vi "Process.vi"(8 "error in":errorcluster, 11 "Logger":refnum<class "Logger.lvclass">) -> (0 "error out":errorcluster, 3 "Logger out":refnum<class "Logger.lvclass">)   [LabVIEW 2019, in "Logger.lvlib" / "Logger.lvclass"]
doc: "---------------------------------------------------------------\nJKI State Machine Objects™\nhttp://jki.net/state-machine-objects/\nCopyright (C) 2005-2015, JKI <info@jki.net>\nALL RIGHTS RESERVED"
uses:
  Logger.lvclass
  C:/Program Files (x86)/National Instruments/LabVIEW 2019/vi.lib/JKI/JKI SMO/smo.lvlibp/SMO/SMO.lvclass
  <vilib>/JKI/JKI SMO/smo.lvlibp/SMO/SMO.lvclass
  <userlib>/LevyLab/Debug/Debug.lvlib
panel:
  out "String":string
  # "For instructions on how to use the JKI State Machine Objects, examples and video tutorials, visit:\nhttp://jki.net/state-machine-objects/\n\nJKI State Machine Objects™\nhttp://jki.net/state-machine-objects/\nCopyright (C) 2005-2015, JKI <info@jki.net>\nALL RIGHTS RESERVED"
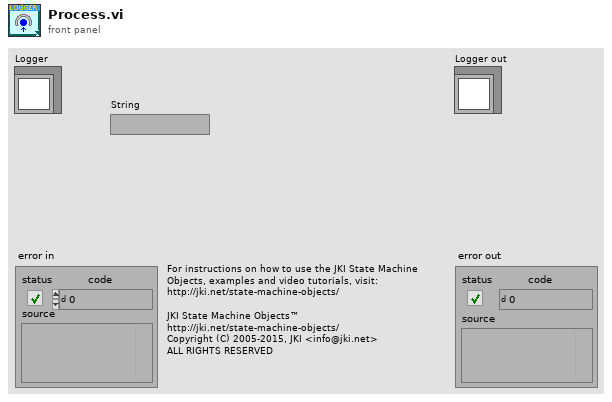
[diagram p1: front panel]
types:
  T1 = enum32{"invalid app kind", "Development System", "Run Time System", "Student Edition", "Embedded LabVIEW", "Evaluation", "Custom"}
  T2 = enum32{"Invalid", "Standard", "Closed", "Hidden", "Minimized", "Maximized"}
  T3 = cluster{"Core":cluster{"Current VI Reference":refnum<vi>, "Close Panel on Exit?":bool, "Last Error":cluster{"error":errorcluster, "previous state":string, "remaining states":string}, "Shutdown?":bool}, "SelfRef":refnum<class "Logger.lvclass">}
  T4 = cluster{"Current VI Reference":refnum<vi>, "Close Panel on Exit?":bool, "Last Error":cluster{"error":errorcluster, "previous state":string, "remaining states":string}, "Shutdown?":bool}
  T5 = typedef "Debug.lvlib/Attribute.Debug.lvclass/DebugBehavior.ctl" = enum16{"Normal", "Debug"}
  T6 = typedef "smo.lvlibp/SMO.lvclass/Protected Events.ctl" = cluster{"StopProcesses":refnum<user-event>, "AbortProcesses":refnum<user-event>, "Config Changed":refnum<user-event>, "Dependency":refnum<user-event>}
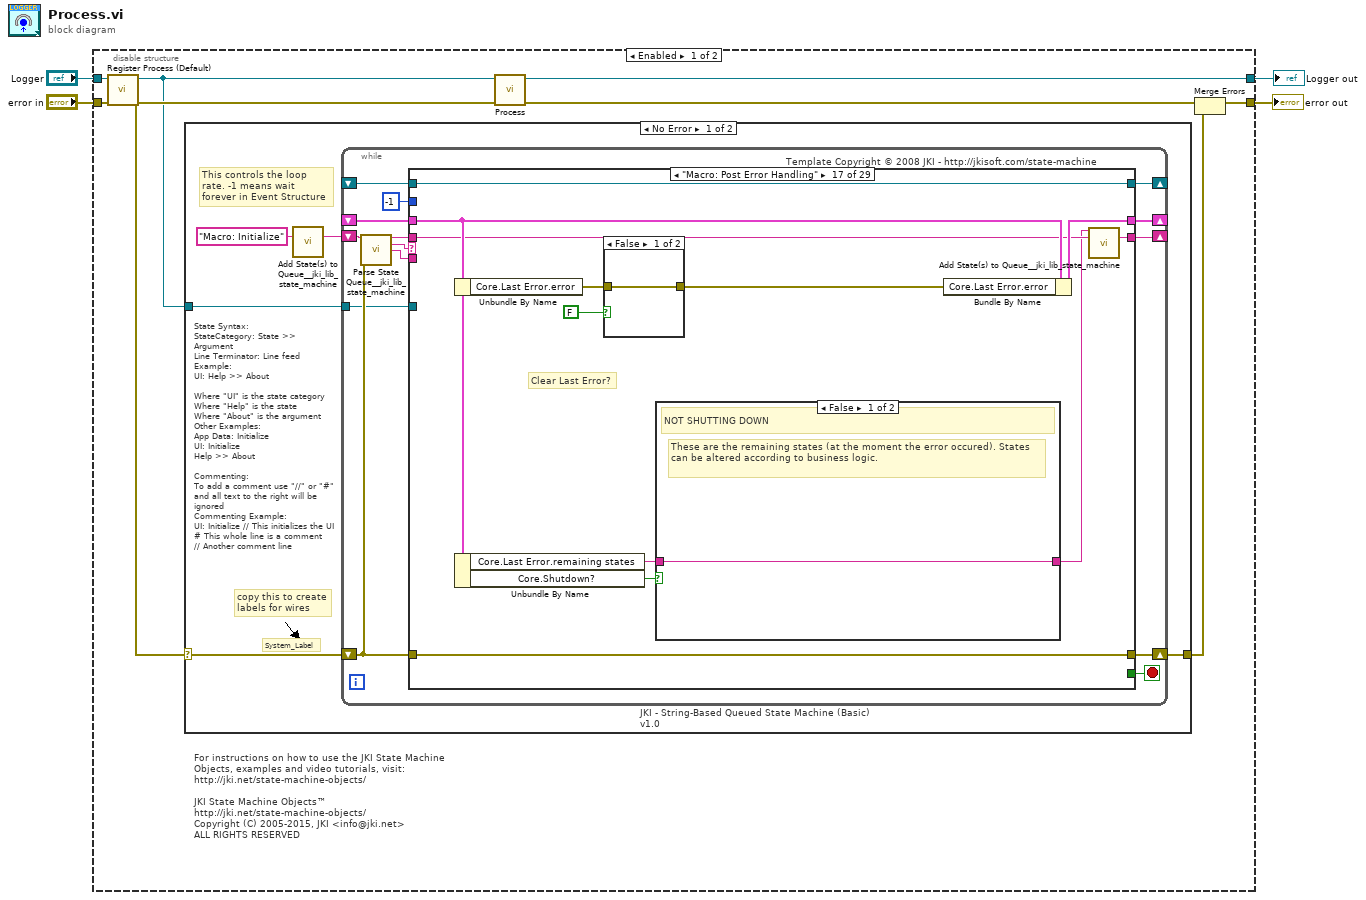
[diagram p0: block diagram]
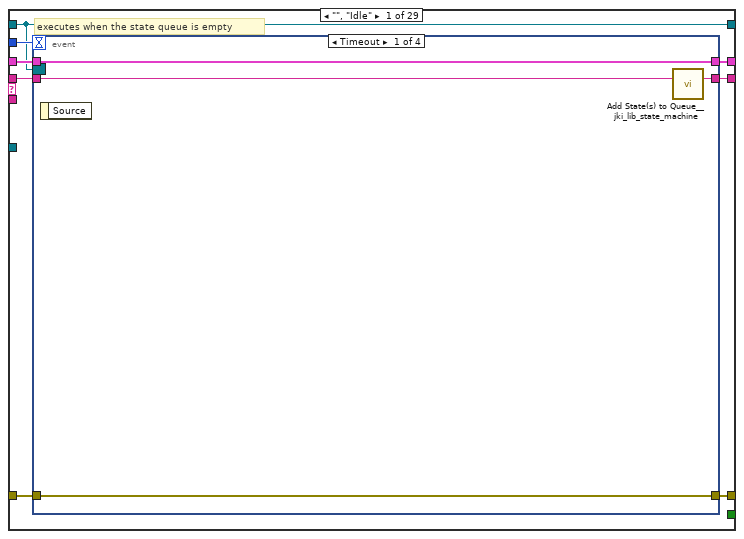
[diagram p2: hidden frame]
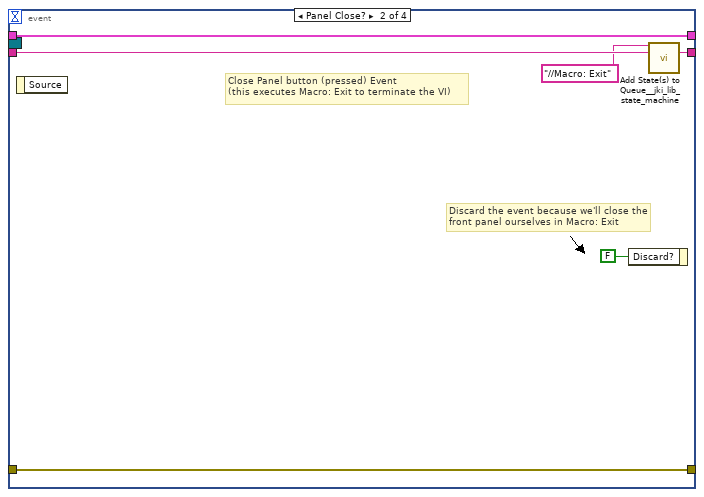
[diagram p3: hidden frame]
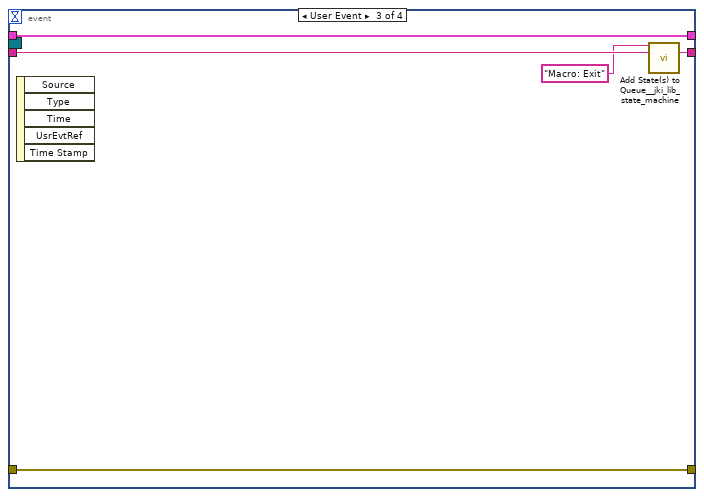
[diagram p4: hidden frame]
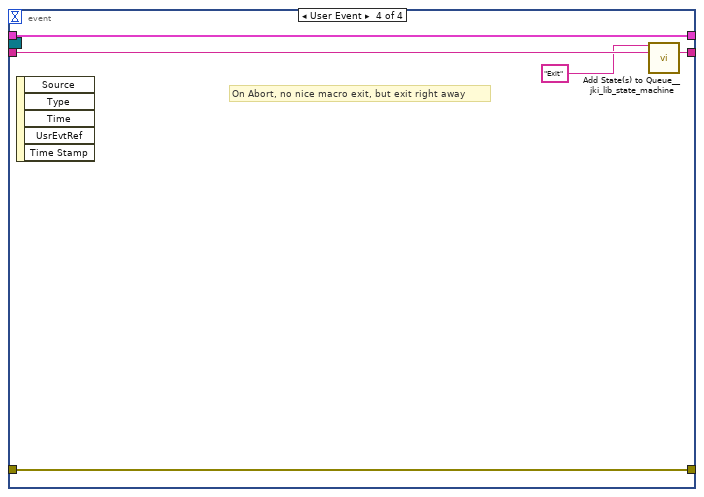
[diagram p5: hidden frame]
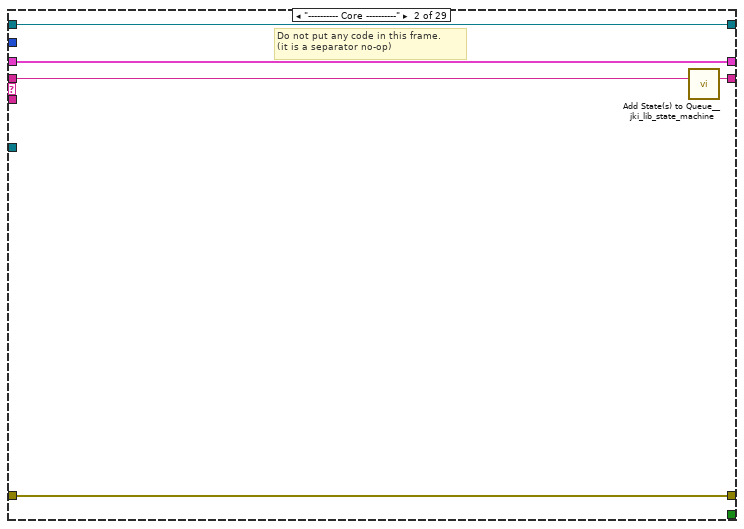
[diagram p6: hidden frame]
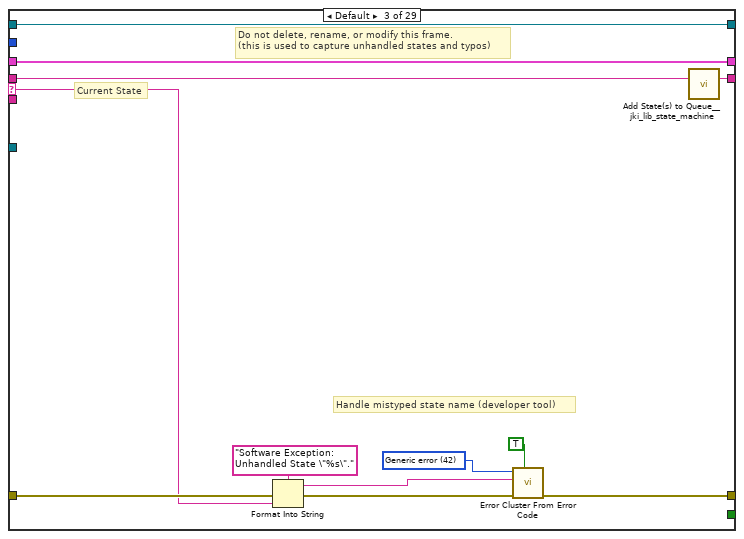
[diagram p7: hidden frame]
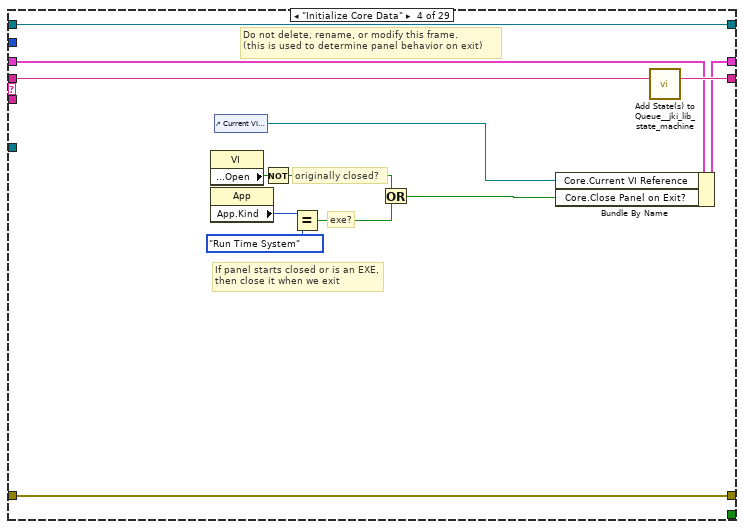
[diagram p8: hidden frame]
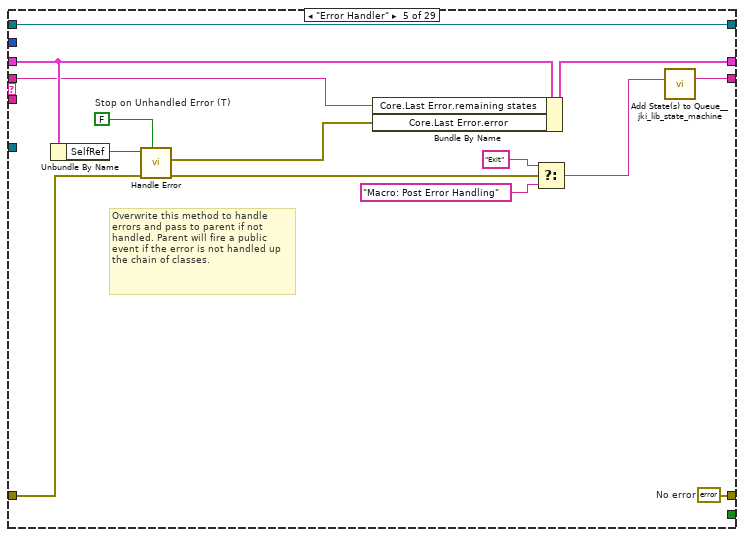
[diagram p9: hidden frame]
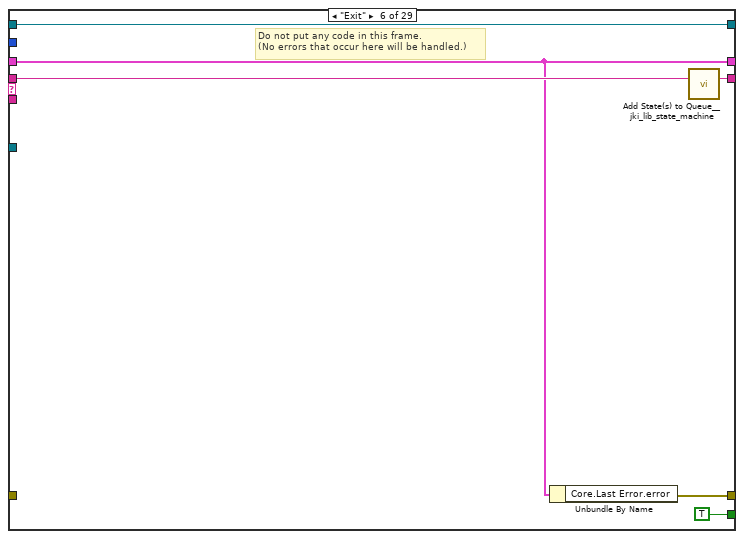
[diagram p10: hidden frame]
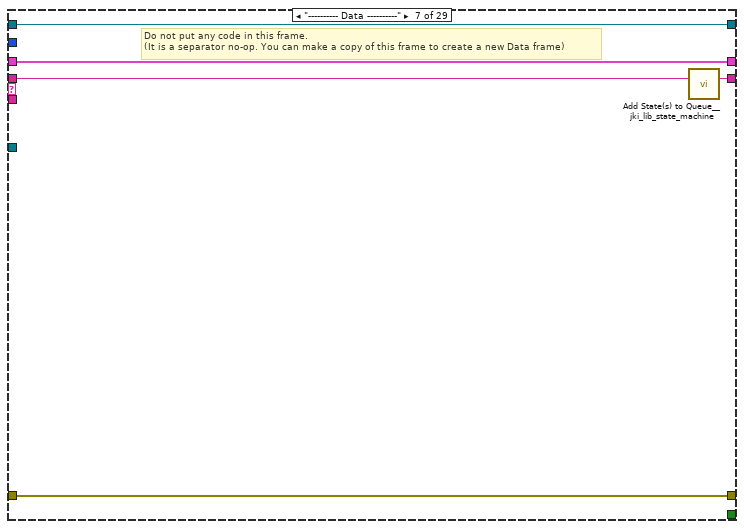
[diagram p11: hidden frame]
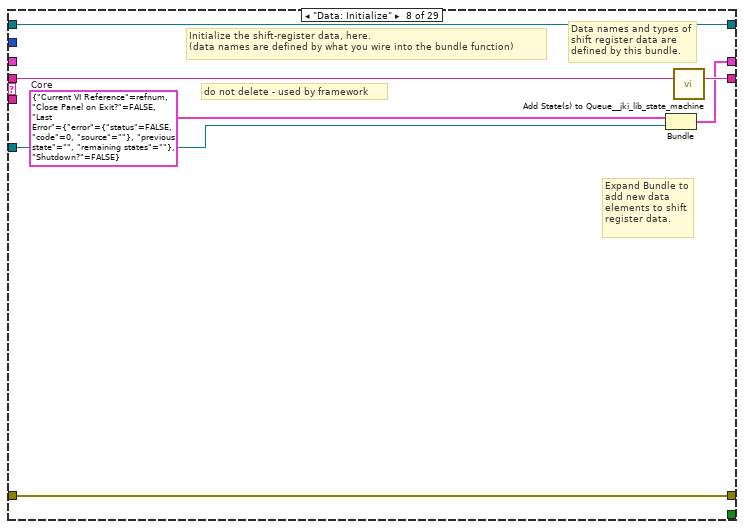
[diagram p12: hidden frame]
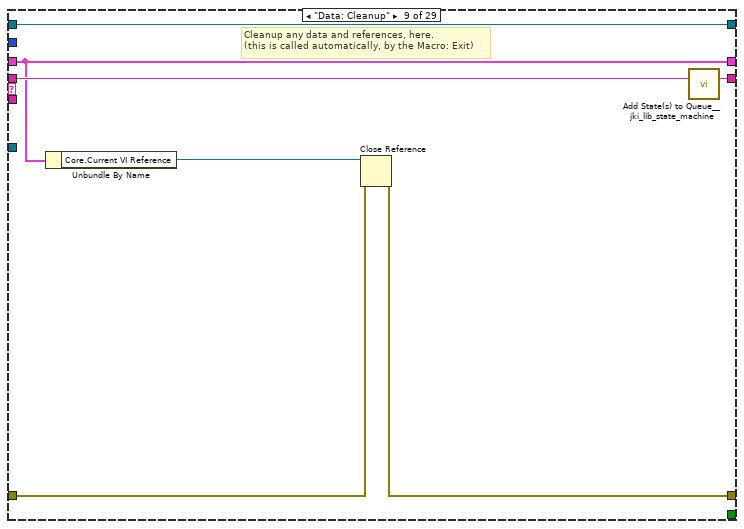
[diagram p13: hidden frame]
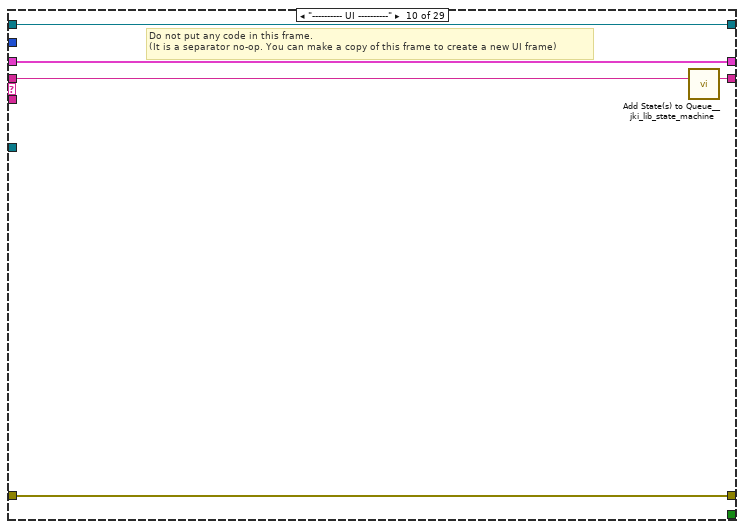
[diagram p14: hidden frame]
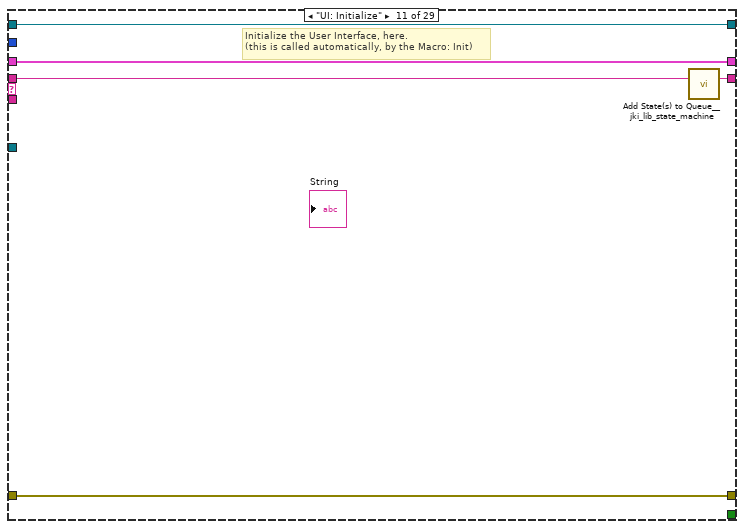
[diagram p15: hidden frame]
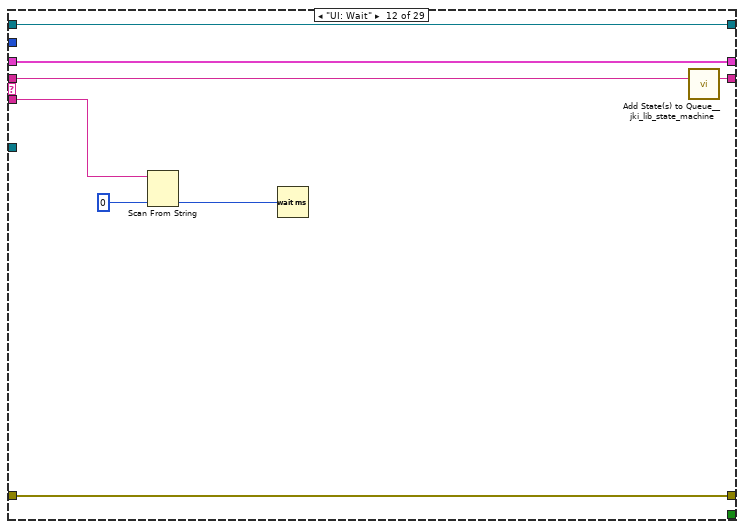
[diagram p16: hidden frame]
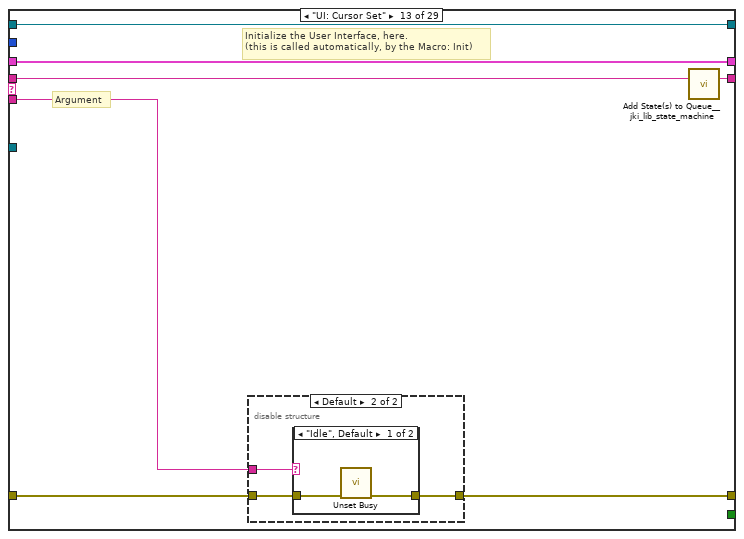
[diagram p17: hidden frame]
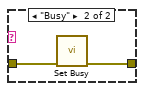
[diagram p19: hidden frame]
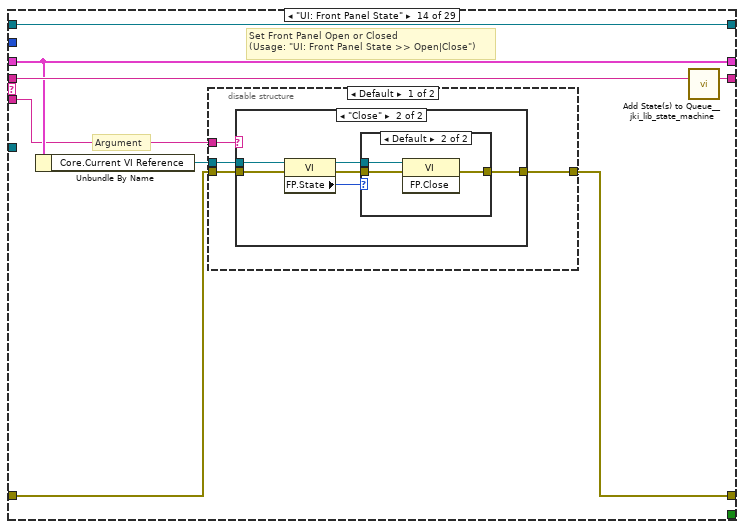
[diagram p20: hidden frame]
diagram:
  n1 = disable-structure shown="Enabled" {
    disable-tunnel: "Logger" -> [w12 w336]
    disable-tunnel: "error in" -> [w11 w335]
    disable-tunnel: [w10 w335] -> w2
    disable-tunnel: [w7 w336] -> w1
    frame Enabled {
      # "For instructions on how to use the JKI State Machine Objects, examples and video tutorials, visit:\nhttp://jki.net/state-machine-objects/\n\nJKI State Machine Objects™\nhttp://jki.net/state-machine-objects/\nCopyright (C) 2005-2015, JKI <info@jki.net>\nALL RIGHTS RESERVED"
      n2 = call <vilib>:"Register Process (Default).vi"("error in (no error)"=w11, "SMO"=w12) -> ("error out"=w9:errorcluster, "SelfRef"=w8:refnum<class "Logger.lvclass">)  [unwired: 8 in]
      n3 = case shown="No Error" w9 {
        selector: w9 -> [w14 w334]
        tunnel: w8 -> [w15 _]
        tunnel: [w13 w334] -> w5
        frame No Error {
          # "State Syntax:\nStateCategory: State >> Argument\nLine Terminator: Line feed\nExample:\nUI: Help >> About\n\nWhere \"UI\" is the state category\nWhere \"Help\" is the state\nWhere \"About\" is the argument\nOther Examples:\nApp Data: Initialize\nUI: Initialize\nHelp >> About\n\nCommenting:\nTo add a comment use \"//\" or \"#\" and all text to the right will be ignored\nCommenting Example:\nUI: Initialize // This initializes the UI\n# This whole line is a comment\n// Another comment line"
          # "copy this to create labels for wires"
          # "This controls the loop rate. -1 means wait forever in Event Structure"
          # "System_Label"
          n4 = call <vilib>:"Add State(s) to Queue__jki_lib_state_machine.vi"("State(s) in (\"\")"="Macro: Initialize") -> ("States Out"=w17:string)  [unwired: 14 in]
          n5 = while "JKI - String-Based Queued State Machine (Basic) v1.0" {
            shift-right: [w19] -> _
            shift-left: _ -> [w18]
            shift-right: [w27] -> w13
            shift-left: w14 -> [w23]
            shift-right: [w26] -> _
            shift-left: w17 -> [w28]
            tunnel: w15 -> [w22]
            shift-right: [w21] -> _
            shift-left: _ -> [w20]
            stop <- w25 stop-if-true
            # "Template Copyright © 2008 JKI - http://jkisoft.com/state-machine"
            n6 = call <vilib>:"Parse State Queue__jki_lib_state_machine.vi"("State Queue"=w28, "Error In (no error)"=w23) -> ("Remaining States"=w30:string, "Current State"=w31:string, "Arguments"=w29:string)  [unwired: 11 in]
            n7 = case shown="\"Macro: Post Error Handling\"" w31 {
              selector: w31 -> [_ _ w66 _ _ _ _ _ _ _ _ _ _ _ _ _ _ _ _ _ _ _ _ _ _ _ _ _ _]
              tunnel: w30 -> [w39 w64 w70 w89 w92 w109 w114 w121 w128 w133 w138 w146 w153 w169 w201 w213 w215 w244 w265 w270 w281 w286 w296 w302 w307 w316 w321 w326 w333]
              tunnel: w29 -> [_ _ _ _ _ _ _ _ _ _ _ w139 w147 w163 _ _ _ _ _ _ _ _ _ _ _ _ _ _ _]
              tunnel: w18 -> [w37 w61 w68 w80 w93 w105 w111 _ w123 w130 w136 w143 w151 w165 w198 w206 w216 w232 w251 w267 w271 w283 w294 w300 w305 w313 w317 w322 w330]
              tunnel: [w36 w62 w72 w86 w99 w104 w112 w115 w124 w131 w135 w144 w148 w166 w199 w202 w224 w231 w263 w268 w273 w284 w289 w298 w303 w308 w318 w323 w327] -> w27
              tunnel: w23 -> [w35 w62 w71 w86 w100 _ w112 w115 w125 w131 w135 w144 w149 w167 w199 w202 w224 w230 w263 w268 w274 w284 w290 w298 w303 w309 w318 w323 w328]
              tunnel: [w38 w63 w69 w88 w103 w108 w113 w120 w127 w132 w137 w145 w152 w168 w200 w212 w225 w243 w264 w269 w280 w285 w295 w301 w306 w315 w320 w325 w332] -> w26
              tunnel: [_ _ _ _ _ TRUE _ _ _ _ _ _ _ _ _ _ _ _ _ _ _ _ _ _ _ _ _ _ _] -> w25
              tunnel: [w34 w61 w68 w87 w98 w105 w111 w117 w123 w130 w136 w143 w151 w165 w198 w206 w217 w234 w252 w267 w271 w283 w294 w300 w305 w312 w317 w322 w330] -> w19
              tunnel: -1 ("Timeout") -> [w33 _ _ _ _ _ _ _ _ _ _ _ _ _ _ _ _ _ _ _ _ _ _ _ _ _ _ _ _]
              tunnel: w22 -> [_ _ _ _ _ _ _ w116 _ _ _ _ _ _ _ _ _ _ _ _ _ _ _ _ _ _ _ _ _]
              tunnel: [w32 w60 w65 w77 w102 w106 w110 w119 w122 w129 w134 w142 w150 w162 w197 w211 w223 w242 w258 w266 w279 w282 w293 w299 w304 w314 w319 w324 w331] -> w21
              tunnel: w20 -> [w32 w60 w65 w77 w102 w106 w110 w119 w122 w129 w134 w142 w150 w162 w197 w211 w223 w242 w258 w266 w279 w282 _ w299 w304 w314 w319 w324 w331]
              frame "", "Idle" {
                # "executes when the state queue is empty"
                n8 = event shown="[0] Timeout" {
                  selector: w32 -> [_ _ _ _]
                  dyn-events: _ -> [_ _ _ _]
                  timeout: w33 -> [_ _ _ _]
                  tunnel: w39 -> [w43 w49 w54 w59]
                  tunnel: [w42 w48 w53 w58] -> w38
                  tunnel: w37 -> [w41 w46 w51 w56]
                  tunnel: [w40 w47 w52 w57] -> w36
                  tunnel: w35 -> [w40 w47 w52 w57]
                  tunnel: [w41 w46 w51 w56] -> w34
                  event Timeout {
                    n9 = event-data() -> ()  [unwired: 1 in, 1 out]
                    n10 = call <vilib>:"Add State(s) to Queue__jki_lib_state_machine.vi"("State(s) in (\"\")"=w43) -> ("States Out"=w42:string)  [unwired: 14 in]
                  }
                  event Panel Close? {
                    # "Discard the event because we'll close the front panel ourselves in Macro: Exit"
                    # "Close Panel button (pressed) Event\n(this executes Macro: Exit to terminate the VI)"
                    n11 = event-data() -> ()  [unwired: 1 in, 1 out]
                    n12 = event-data("Discard?"=FALSE) -> ()  [unwired: 1 in, 1 out]
                    n13 = call <vilib>:"Add State(s) to Queue__jki_lib_state_machine.vi"("State(s) in Front (\"\")"="//Macro: Exit", "State(s) in (\"\")"=w49) -> ("States Out"=w48:string)  [unwired: 13 in]
                  }
                  event User Event {
                    n14 = event-data() -> ()  [unwired: 1 in, 5 out]
                    n15 = call <vilib>:"Add State(s) to Queue__jki_lib_state_machine.vi"("State(s) in Front (\"\")"="Macro: Exit", "State(s) in (\"\")"=w54) -> ("States Out"=w53:string)  [unwired: 13 in]
                  }
                  event User Event {
                    # "On Abort, no nice macro exit, but exit right away"
                    n16 = event-data() -> ()  [unwired: 1 in, 5 out]
                    n17 = call <vilib>:"Add State(s) to Queue__jki_lib_state_machine.vi"("State(s) in Front (\"\")"="Exit", "State(s) in (\"\")"=w59) -> ("States Out"=w58:string)  [unwired: 13 in]
                  }
                }
              }
              frame "---------- Core ----------" {
                # "Do not put any code in this frame.\n(it is a separator no-op)"
                n18 = call <vilib>:"Add State(s) to Queue__jki_lib_state_machine.vi"("State(s) in (\"\")"=w64) -> ("States Out"=w63:string)  [unwired: 14 in]
              }
              frame Default {
                w75 = 42 items=["No error", "Argument error", "Memory is full", "Out of zone", "End of file", "File already open", "Generic file I/O error", "File not found", "File permission error", "Disk is full", "Duplicate path", "Too many files open", "System feature not enabled", "Resource file not found", "Cannot add resource", "Resource not found", "Image not found", "Image memory error", "Pen does not exist", "Config type invalid", "Config token not found", "Config parse error", "Config memory error", "Bad external code format", "Bad external code offset", "External code not present", "Null window", "Destroy window error", "Null menu", "Print aborted", "Bad print record", "Print driver error", "Windows error during printing", "Memory error during printing", "Print dialog error", "Generic print error", "Invalid device refnum", "Device not found", "Device parameter error", "Device unit error", "Cannot open device", "Device call aborted", "Generic error", "Cancelled by user", "Object ID too low", "Object ID too high", "Object not in heap", "Unknown heap", "Unknown object (invalid DefProc)", "Unknown object (DefProc not in table)", "Message out of range", "Invalid (null) method", "Unknown message", "Manager call not supported", "Bad address", "Network operation in progress", "Network operation timed out", "Connection is busy", "Network attribute not supported", "Network error", "Address in use", "System out of memory", "Connection aborted", "Connection refused", "Not connected", "Already connected", "Connection closed", "Initialization error (interapplication manager)", "Bad occurrence", "Wait on unbound occurrence handler", "Occurrence queue overflow", "Datalog type conflict", "Unused", "Unrecognized type (interapplication manager)", "Memory corrupt", "Failed to make temporary DLL", "Old CIN version", "Drag socket not found", "Failed to load drop-object", "Failed to register OLE object", "Failed to release OLE object", "Format specifier type mismatch", "Unknown format specifier", "Too few format specifiers", "Too many format specifiers", "Scan failed", "Newer CIN version", "Error converting to variant", "Runtime menu error", "Password tampered", "Variant attribute not found", "Incompatible variant data type", "Event data is not available", "Event Store is not present", "Occurrence is not found", "Event Queue is not created", "Event info is not available", "Refnum passed is NULL", "Error retrieving Class GUID", "Error retrieving CoClass GUID", "Error retrieving TypeLib GUID.", "Bad built application magic bytes.", "Specific driver is different from the specific driver associated with the Logical Name.", "There is no session opened to the class driver.", "Max Error", "MAX - Error with config objects", "MAX - Error loading configuration", "MAX - Group not supported"]
                # "Current State"
                # "Do not delete, rename, or modify this frame.\n(this is used to capture unhandled states and typos)"
                # "Handle mistyped state name (developer tool)"
                n19 = Format Into String(format string="Software Exception: Unhandled State \"%s\"." ("message"), error in=w71, w66) -> (resulting string=w74:string, error out=w73:errorcluster)  [unwired: 1 in]
                n20 = call <vilib>:"Error Cluster From Error Code.vi"("show call chain? (False)"=TRUE, "error in (no error)"=w73, "error message (\"\")"=w74, "error code (0)"=w75) -> ("error out"=w72:errorcluster)  [unwired: 5 in]
                n21 = call <vilib>:"Add State(s) to Queue__jki_lib_state_machine.vi"("State(s) in (\"\")"=w70) -> ("States Out"=w69:string)  [unwired: 14 in]
              }
              frame "Initialize Core Data" {
                # "Do not delete, rename, or modify this frame.\n(this is used to determine panel behavior on exit)"
                # "originally closed?"
                # "exe?"
                # "If panel starts closed or is an EXE, then close it when we exit"
                n22 = property class="VI"() -> ("Front Panel.Open"=w85:bool)  [unwired: 2 in, 2 out]
                n23 = property class="App"() -> ("App.Kind"=w84:T1)  [unwired: 2 in, 2 out]
                n24 = control-ref of="Current VI Reference"() -> (w78:refnum<vi>)
                n25 = Not(x=w85) -> (.not. x?=w82:bool)
                n26 = Equal?(x=w84, y=T1."Run Time System" ("Application:Kind")) -> (x = y?=w81:bool)
                n27 = Or(x=w82, y=w81) -> (x .or. y?=w79:bool)
                n28 = Bundle By Name(cluster=w80, "Core.Current VI Reference"=w78, "Core.Close Panel on Exit?"=w79) -> (w87:T3)
                n29 = call <vilib>:"Add State(s) to Queue__jki_lib_state_machine.vi"("State(s) in (\"\")"=w89) -> ("States Out"=w88:string)  [unwired: 14 in]
              }
              frame "Error Handler" {
                w94 = FALSE  # Stop on Unhandled Error (T)
                w99 = errorcluster {"status"=FALSE, "code"=0, "source"=""}  # No error
                # "Overwrite this method to handle errors and pass to parent if not handled. Parent will fire a public event if the error is not handled up the chain of classes."
                n30 = Unbundle By Name(w93) -> ("SelfRef"=w101:refnum<class "Logger.lvclass">)
                n31 = call-dynamic "Handle Error.vi"("Stop on Unhandled Error (T)"=w94, "error in"=w100, "SMO"=w101) -> ("handling error"=w95:errorcluster, "Unhandled error"=w97:errorcluster)  [unwired: 6 in, 1 out]
                n32 = Bundle By Name(cluster=w93, "Core.Last Error.remaining states"=w92, "Core.Last Error.error"=w97) -> (w98:T3)
                n33 = Select(t="Exit", s=w95, f="Macro: Post Error Handling") -> (s? t:f=w90:string)
                n34 = call <vilib>:"Add State(s) to Queue__jki_lib_state_machine.vi"("State(s) in (\"\")"=w90) -> ("States Out"=w103:string)  [unwired: 14 in]
              }
              frame "Exit" {
                # "Do not put any code in this frame.\n(No errors that occur here will be handled.)"
                n35 = Unbundle By Name(w105) -> ("Core.Last Error.error"=w104:errorcluster)
                n36 = call <vilib>:"Add State(s) to Queue__jki_lib_state_machine.vi"("State(s) in (\"\")"=w109) -> ("States Out"=w108:string)  [unwired: 14 in]
              }
              frame "---------- Data ----------" {
                # "Do not put any code in this frame.\n(It is a separator no-op. You can make a copy of this frame to create a new Data frame)"
                n37 = call <vilib>:"Add State(s) to Queue__jki_lib_state_machine.vi"("State(s) in (\"\")"=w114) -> ("States Out"=w113:string)  [unwired: 14 in]
              }
              frame "Data: Initialize" {
                w118 = T4 {"Current VI Reference"=refnum, "Close Panel on Exit?"=FALSE, "Last Error"={"error"={"status"=FALSE, "code"=0, "source"=""}, "previous state"="", "remaining states"=""}, "Shutdown?"=FALSE}  # Core
                # "do not delete - used by framework"
                # "Expand Bundle to add new data elements to shift register data."
                # "Data names and types of shift register data are defined by this bundle."
                # "Initialize the shift-register data, here.\n(data names are defined by what you wire into the bundle function)"
                n38 = Bundle("Core"=w118, "SelfRef"=w116) -> (w117:T3)  [unwired: 1 in]
                n39 = call <vilib>:"Add State(s) to Queue__jki_lib_state_machine.vi"("State(s) in (\"\")"=w121) -> ("States Out"=w120:string)  [unwired: 14 in]
              }
              frame "Data: Cleanup" {
                # "Cleanup any data and references, here.\n(this is called automatically, by the Macro: Exit)"
                n40 = Unbundle By Name(w123) -> ("Core.Current VI Reference"=w126:refnum<vi>)
                n41 = Close Reference(reference=w126, error in (no error)=w125) -> (error out=w124:errorcluster)
                n42 = call <vilib>:"Add State(s) to Queue__jki_lib_state_machine.vi"("State(s) in (\"\")"=w128) -> ("States Out"=w127:string)  [unwired: 14 in]
              }
              frame "---------- UI ----------" {
                # "Do not put any code in this frame.\n(It is a separator no-op. You can make a copy of this frame to create a new UI frame)"
                n43 = call <vilib>:"Add State(s) to Queue__jki_lib_state_machine.vi"("State(s) in (\"\")"=w133) -> ("States Out"=w132:string)  [unwired: 14 in]
              }
              frame "UI: Initialize" {
                # "Initialize the User Interface, here.\n(this is called automatically, by the Macro: Init)"
                n44 = call <vilib>:"Add State(s) to Queue__jki_lib_state_machine.vi"("State(s) in (\"\")"=w138) -> ("States Out"=w137:string)  [unwired: 14 in]
              }
              frame "UI: Wait" {
                n45 = Scan From String(input string=w139, default 1=u32 0) -> (output 1=w140:u32)  [unwired: 3 in, 3 out]
                n46 = Wait (ms)(milliseconds to wait=w140) -> ()  [unwired: 1 out]
                n47 = call <vilib>:"Add State(s) to Queue__jki_lib_state_machine.vi"("State(s) in (\"\")"=w146) -> ("States Out"=w145:string)  [unwired: 14 in]
              }
              frame "UI: Cursor Set" {
                # "Argument"
                # "Initialize the User Interface, here.\n(this is called automatically, by the Macro: Init)"
                n48 = disable-structure shown="Default" {
                  disable-tunnel: w149 -> [w154 w157]
                  disable-tunnel: [w154 w156] -> w148
                  disable-tunnel: w147 -> [_ w155]
                  frame condition #0 {
                  }
                  frame condition #1 (active) {
                    n49 = case shown="\"Idle\", Default" w155 {
                      tunnel: w157 -> [w159 w161]
                      tunnel: [w158 w160] -> w156
                      frame "Idle", Default {
                        n50 = call <vilib>:"Unset Busy.vi"("error in (no error)"=w159) -> ("error out"=w158:errorcluster)  [unwired: 10 in]
                      }
                      frame "Busy" {
                        n51 = call <vilib>:"Set Busy.vi"("error in (no error)"=w161) -> ("error out"=w160:errorcluster)  [unwired: 9 in, 1 out]
                      }
                    }
                  }
                }
                n52 = call <vilib>:"Add State(s) to Queue__jki_lib_state_machine.vi"("State(s) in (\"\")"=w153) -> ("States Out"=w152:string)  [unwired: 14 in]
              }
              frame "UI: Front Panel State" {
                # "Argument"
                # "Set Front Panel Open or Closed\n(Usage: \"UI: Front Panel State >> Open|Close\")"
                n53 = Unbundle By Name(w165) -> ("Core.Current VI Reference"=w164:refnum<vi>)
                n54 = disable-structure shown="Default" {
                  disable-tunnel: w167 -> [w173 w196]
                  disable-tunnel: [w172 w196] -> w166
                  disable-tunnel: w164 -> [w171 _]
                  disable-tunnel: w163 -> [w170 _]
                  frame condition #0 (active) {
                    n55 = case shown="\"Close\"" w170 {
                      tunnel: w173 -> [w177 w190]
                      tunnel: [w179 w191] -> w172
                      tunnel: w171 -> [w178 w188]
                      frame "Open", Default {
                        n56 = property class="VI"(reference=w178, error in=w177) -> (reference out=w175:refnum<vi>, error out=w176:errorcluster, "FP.State"=w174:T2)
                        n57 = case shown="\"Closed\"" w174 {
                          tunnel: [w182 w185] -> w179
                          tunnel: w176 -> [w181 w185]
                          tunnel: w175 -> [w180 _]
                          frame "Closed" {
                            n58 = invoke class="VI" method="FP.Open"(reference=w180, error in=w181, "Activate"=TRUE, "State"=T2."Standard") -> (error out=w182:errorcluster)  [unwired: 1 in, 4 out]
                          }
                          frame Default {
                          }
                        }
                      }
                      frame "Close" {
                        n59 = property class="VI"(reference=w188, error in=w190) -> (reference out=w187:refnum<vi>, error out=w189:errorcluster, "FP.State"=w186:T2)
                        n60 = case shown="Default" w186 {
                          tunnel: [w192 w195] -> w191
                          tunnel: w189 -> [w192 w194]
                          tunnel: w187 -> [_ w193]
                          frame "Invalid", "Closed" {
                          }
                          frame Default {
                            n61 = invoke class="VI" method="FP.Close"(reference=w193, error in=w194) -> (error out=w195:errorcluster)  [unwired: 1 in, 2 out]
                          }
                        }
                      }
                    }
                  }
                  frame condition #1 {
                  }
                }
                n62 = call <vilib>:"Add State(s) to Queue__jki_lib_state_machine.vi"("State(s) in (\"\")"=w169) -> ("States Out"=w168:string)  [unwired: 14 in]
              }
              frame "---------- Macro ----------" {
                # "Do not put any code in this frame.\n(It is a separator no-op. You can make a copy of this frame to create a new Macro frame)"
                n63 = call <vilib>:"Add State(s) to Queue__jki_lib_state_machine.vi"("State(s) in (\"\")"=w201) -> ("States Out"=w200:string)  [unwired: 14 in]
              }
              frame "Macro: Initialize" {
                # "Initialization Macro\n(This is called once, when the VI starts)"
                n64 = call <vilib>:"Add State(s) to Queue__jki_lib_state_machine.vi"("State(s) in Front (\"\")"="", "State(s) in (\"\")"="UI: Initialize\nUI: Front Panel State >> Close", "State(s) at Back (\"\")"="Macro: Debug\nLogger: Create Logger") -> ("States Out"=w207:string)  [unwired: 12 in]
                n65 = call <vilib>:"Add State(s) to Queue__jki_lib_state_machine.vi"("State(s) in Front (\"\")"="Data: Initialize\nInitialize Core Data\nEvents: Register", "State(s) in (\"\")"="Process: Sync", "State(s) at Back (\"\")"=w207) -> ("States Out"=w209:string)  [unwired: 12 in]
                n66 = call <vilib>:"Add State(s) to Queue__jki_lib_state_machine.vi"("State(s) in Front (\"\")"=w209, "State(s) in (\"\")"=w213) -> ("States Out"=w212:string)  [unwired: 13 in]
              }
              frame "Macro: Post Error Handling" {
                # "Clear Last Error?"
                n67 = Unbundle By Name(w216) -> ("Core.Last Error.error"=w220:errorcluster)
                n68 = Unbundle By Name(w216) -> ("Core.Last Error.remaining states"=w222:string, "Core.Shutdown?"=w221:bool)
                n69 = case shown="False" FALSE {
                  tunnel: w220 -> [w226 _]
                  tunnel: [w226 _] -> w218
                  frame False {
                  }
                  frame True {
                  }
                }
                n70 = case shown="False" w221 {
                  tunnel: w222 -> [w227 w229]
                  tunnel: [w227 w228] -> w214
                  frame False {
                    # "These are the remaining states (at the moment the error occured). States can be altered according to business logic."
                    # "NOT SHUTTING DOWN"
                  }
                  frame True {
                    # "Developer can decide to alter the states but should be aware that during the shutdown process, there are certain states that must be run for the SMO to properly shut itself (and this process) down. As such, one can add states to perform additional clean-ups, but should append the remaining state to be executed."
                    # "SHUTTING DOWN"
                    n71 = call <vilib>:"Add State(s) to Queue__jki_lib_state_machine.vi"("State(s) in (\"\")"=w229) -> ("States Out"=w228:string)  [unwired: 14 in]
                  }
                }
                n72 = Bundle By Name(cluster=w216, "Core.Last Error.error"=w218) -> (w217:T3)
                n73 = call <vilib>:"Add State(s) to Queue__jki_lib_state_machine.vi"("State(s) in Front (\"\")"=w214, "State(s) in (\"\")"=w215) -> ("States Out"=w225:string)  [unwired: 13 in]
              }
              frame "Macro: Debug" {
                # "exe?"
                # "If pane is an EXE, then close it when we exit"
                # "Macro: Debug\n(get debug behavior, determine UI and determine shutdown behavior)"
                n74 = Unbundle By Name(w232) -> ("Core.Close Panel on Exit?"=w236:bool, "SelfRef"=w241:refnum<class "Logger.lvclass">)
                n75 = property class="App"() -> ("App.Kind"=w239:T1)  [unwired: 2 in, 2 out]
                n76 = Equal?(x=w239, y=T1."Run Time System" ("Application:Kind")) -> (x = y?=w235:bool)
                n77 = call <userlib>:"Get Debug Mode.vi"("error in (no error)"=w230, "SMO"=w241) -> ("error out"=w231:errorcluster, "Behavior"=w240:T5)  [unwired: 7 in, 1 out]
                n78 = case shown="\"Debug\"" w240 {
                  tunnel: [_ "UI: Front Panel State >> Open\nUI: Wait >> 1000"] -> w233
                  tunnel: [w245 w246] -> w237
                  tunnel: w236 -> [w245 _]
                  tunnel: w235 -> [_ w248]
                  frame "Normal", Default {
                    # "respect core.close"
                  }
                  frame "Debug" {
                    # "keep panel open\nunless exe"
                    n79 = Or(x=w248, y=FALSE) -> (x .or. y?=w246:bool)
                  }
                }
                n80 = Bundle By Name(cluster=w232, "Core.Close Panel on Exit?"=w237) -> (w234:T3)
                n81 = call <vilib>:"Add State(s) to Queue__jki_lib_state_machine.vi"("State(s) in Front (\"\")"=w233, "State(s) in (\"\")"=w244) -> ("States Out"=w243:string)  [unwired: 13 in]
              }
              frame "Macro: Exit" {
                # "Exit Macro\n(This is called once, when the VI exits)"
                n82 = Unbundle By Name(w251) -> ("Core.Close Panel on Exit?"=w262:bool)
                n83 = Bundle By Name(cluster=w251, "Core.Shutdown?"=TRUE) -> (w252:T3)
                n84 = Select(t="UI: Front Panel State >> Close", s=w262, f="") -> (s? t:f=w260:string)
                n85 = call <vilib>:"Add State(s) to Queue__jki_lib_state_machine.vi"("State(s) in Front (\"\")"="Logger: Destroy Logger\nData: Cleanup\nEvents: Unregister", "State(s) in (\"\")"="Process: Sync", "State(s) at Back (\"\")"="Exit") -> ("States Out"=w255:string)  [unwired: 12 in]
                n86 = call <vilib>:"Add State(s) to Queue__jki_lib_state_machine.vi"("State(s) in (\"\")"=w260, "State(s) at Back (\"\")"=w255) -> ("States Out"=w259:string)  [unwired: 13 in]
                n87 = call <vilib>:"Add State(s) to Queue__jki_lib_state_machine.vi"("State(s) in Front (\"\")"=w259, "State(s) in (\"\")"=w265) -> ("States Out"=w264:string)  [unwired: 13 in]
              }
              frame "---------- Process ----------" {
                # "Template Separator\n(You can make a copy of, or modify, this frame)"
                n88 = call <vilib>:"Add State(s) to Queue__jki_lib_state_machine.vi"("State(s) in (\"\")"=w270) -> ("States Out"=w269:string)  [unwired: 14 in]
              }
              frame "Process: Sync" {
                n89 = Unbundle By Name(w271) -> ("SelfRef"=w275:refnum<class "Logger.lvclass">)
                n90 = call <vilib>:"WaitOnProcessSync.vi"("error in (no error)"=w274, "SMO"=w275) -> ("error out"=w273:errorcluster, "Don't run?"=w278:bool)  [unwired: 7 in, 1 out]
                n91 = Select(t="Data: Cleanup\nEvents: Unregister\nExit", s=w278, f="") -> (s? t:f=w272:string)
                n92 = call <vilib>:"Add State(s) to Queue__jki_lib_state_machine.vi"("State(s) in Front (\"\")"=w272, "State(s) in (\"\")"=w281) -> ("States Out"=w280:string)  [unwired: 13 in]
              }
              frame "---------- Events ----------" {
                # "Template Separator\n(You can make a copy of, or modify, this frame)"
                n93 = call <vilib>:"Add State(s) to Queue__jki_lib_state_machine.vi"("State(s) in (\"\")"=w286) -> ("States Out"=w285:string)  [unwired: 14 in]
              }
              frame "Events: Register" {
                # "Expand to add\nmore events"
                n94 = Unbundle By Name(w294) -> ("SelfRef"=w291:refnum<class "Logger.lvclass">)
                n95 = call <vilib>:"GetProtectedEvents.vi"("SMO"=w291) -> ("error out"=w287:errorcluster, "SMO Protected Events"=w292:T6)  [unwired: 8 in, 1 out]
                n96 = register-events(w292) -> (reference out=w293:refnum<event-registration>, error out=w288:errorcluster)  [unwired: 2 in]
                n97 = Merge Errors(w290, w288, w287) -> (w289:errorcluster)
                n98 = call <vilib>:"Add State(s) to Queue__jki_lib_state_machine.vi"("State(s) in (\"\")"=w296) -> ("States Out"=w295:string)  [unwired: 14 in]
              }
              frame "Events: Unregister" {
                n99 = Unregister For Events(event registration refnum=w299, error in=w298) -> (error out=w297:errorcluster)
                n100 = call <vilib>:"Clear Errors.vi"("error in (no error)"=w297) -> ()  [unwired: 5 in, 2 out]
                n101 = call <vilib>:"Add State(s) to Queue__jki_lib_state_machine.vi"("State(s) in (\"\")"=w302) -> ("States Out"=w301:string)  [unwired: 14 in]
              }
              frame "---------- Logger ----------" {
                n102 = call <vilib>:"Add State(s) to Queue__jki_lib_state_machine.vi"("State(s) in (\"\")"=w307) -> ("States Out"=w306:string)  [unwired: 14 in]
              }
              frame "Logger: Create Logger" {
                n103 = Unbundle By Name(w313) -> ("SelfRef"=w311:refnum<class "Logger.lvclass">)
                n104 = call-dynamic "Create Logger.vi"("error in (no error)"=w309, "Logger in"=w311) -> ("error out"=w308:errorcluster, "Logger out"=w310:refnum<class "Logger.lvclass">)  [unwired: 8 in]
                n105 = Bundle By Name(cluster=w313, "SelfRef"=w310) -> (w312:T3)
                n106 = call <vilib>:"Add State(s) to Queue__jki_lib_state_machine.vi"("State(s) in (\"\")"=w316) -> ("States Out"=w315:string)  [unwired: 14 in]
              }
              frame "Logger: Write Logger" {
                n107 = Unbundle By Name(w317) -> ()  [unwired: 1 out]
                n108 = call <vilib>:"Add State(s) to Queue__jki_lib_state_machine.vi"("State(s) in (\"\")"=w321) -> ("States Out"=w320:string)  [unwired: 14 in]
              }
              frame "Logger: Read Logger" {
                n109 = Unbundle By Name(w322) -> ()  [unwired: 1 out]
                n110 = call <vilib>:"Add State(s) to Queue__jki_lib_state_machine.vi"("State(s) in (\"\")"=w326) -> ("States Out"=w325:string)  [unwired: 14 in]
              }
              frame "Logger: Destroy Logger" {
                n111 = Unbundle By Name(w330) -> ("SelfRef"=w329:refnum<class "Logger.lvclass">)
                n112 = call-dynamic "Destroy Logger.vi"("error in (no error)"=w328, "Logger in"=w329) -> ("error out"=w327:errorcluster)  [unwired: 8 in, 1 out]
                n113 = call <vilib>:"Add State(s) to Queue__jki_lib_state_machine.vi"("State(s) in (\"\")"=w333) -> ("States Out"=w332:string)  [unwired: 14 in]
              }
            }
          }
        }
        frame Error {
        }
      }
      n114 = call-parent "Process.vi"("error in"=w9, "SMO"=w8) -> ("error out"=w6:errorcluster, "SMO out"=w7:refnum<class "Logger.lvclass">)  [unwired: 8 in]
      n115 = Merge Errors(w6, w5) -> (w10:errorcluster)
    }
    frame Disabled {
    }
  }
  "Logger out" <- w1
  "error out" <- w2
